vi "Define tração 90°C suporte.vi"(8 "error in (no error)":errorcluster, 11 "Dados SP":T1={"Condutor"={"Pc (N/m)"=0.0, "Mod.Young (N/m²)"=0.0, "Dil.Term.c (m/°C)"=0.0, "Área  (m²)"=0.0, "Tração EDS (N)"=0.0, "Tração Torig(N)"=0.0, "Tração Talta (N)"=0.0}, "Suporte"={"Ps (N/m)"=0.0, "Es (N/m²)"=0.0, "DTc (1/°C)"=0.0, "Área sup (m²)"=0.0, "Tração EDS sup (N)"=0.0, "Tração AT sup (N)"=0.0, "Flecha sup AT (m)"=0.0}, "Vão"={"Extensão (m)"=0.0, "Desnivel (m)"=0.0, "Flecha à 60 °C"=0.0}, "Projeto"={"Temp. EDS (°C)"=0.0, "Lim.original (°C)"=0.0, "Lim.extend. (°C)"=0.0, "N. cabo/fase"=1.0}, "Subvão"={"Ext.Lim (m)"=0.0, "N. Esp."=0.0, "F.lim (m)"=0.0, "Ext.calc"=0.0, "Ext.definido"=0.0, "Comp.cabo"=0.0, "Ext.55%"=0.0, "Tração sub\nAT (N)"=0.0, "Ext.sel."=0.0, "Flecha lim.\ncalc (m)"=0.0}, "Vetor de dados"={"Coor.X.esp"=[], "Coor.Y.Esp."=[], "Sub.vao X"=[], "Sub.vao Y"=[], "CoordY.sup"=[], "CoordX.sup"=[]}} {"Subvão"."Comp.cabo" min=1.0 max=8.0 step=1.0}) -> (0 "error out":errorcluster, 3 "Dados SP Out":T1={"Condutor"={"Pc (N/m)"=0.0, "Mod.Young (N/m²)"=0.0, "Dil.Term.c (m/°C)"=0.0, "Área  (m²)"=0.0, "Tração EDS (N)"=0.0, "Tração Torig(N)"=0.0, "Tração Talta (N)"=0.0}, "Suporte"={"Ps (N/m)"=0.0, "Es (N/m²)"=0.0, "DTc (1/°C)"=0.0, "Área sup (m²)"=0.0, "Tração EDS sup (N)"=0.0, "Tração AT sup (N)"=0.0, "Flecha sup AT (m)"=0.0}, "Vão"={"Extensão (m)"=0.0, "Desnivel (m)"=0.0, "Flecha à 60 °C"=0.0}, "Projeto"={"Temp. EDS (°C)"=0.0, "Lim.original (°C)"=0.0, "Lim.extend. (°C)"=0.0, "N. cabo/fase"=1.0}, "Subvão"={"Ext.Lim (m)"=0.0, "N. Esp."=0.0, "F.lim (m)"=0.0, "Ext.calc"=0.0, "Ext.definido"=0.0, "Comp.cabo"=0.0, "Ext.55%"=0.0, "Tração sub\nAT (N)"=0.0, "Ext.sel."=0.0, "Flecha lim.\ncalc (m)"=0.0}, "Vetor de dados"={"Coor.X.esp"=[], "Coor.Y.Esp."=[], "Sub.vao X"=[], "Sub.vao Y"=[], "CoordY.sup"=[], "CoordX.sup"=[]}} {"Subvão"."Comp.cabo" min=1.0 max=8.0 step=1.0})   [LabVIEW 2020]
uses:
  controls/SP data.ctl
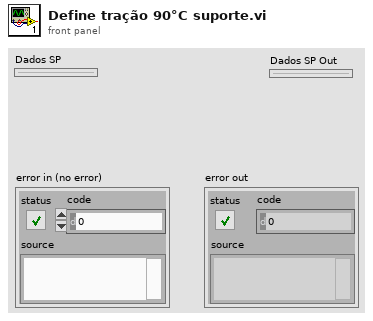
[diagram p1: front panel]
types:
  T1 = typedef "SP data.ctl" = cluster{"Condutor":cluster{"Pc (N/m)":dbl, "Mod.Young (N/m²)":dbl, "Dil.Term.c (m/°C)":dbl, "Área  (m²)":dbl, "Tração EDS (N)":dbl, "Tração Torig(N)":dbl, "Tração Talta (N)":dbl}, "Suporte":cluster{"Ps (N/m)":dbl, "Es (N/m²)":dbl, "DTc (1/°C)":dbl, "Área sup (m²)":dbl, "Tração EDS sup (N)":dbl, "Tração AT sup (N)":dbl, "Flecha sup AT (m)":dbl}, "Vão":cluster{"Extensão (m)":dbl, "Desnivel (m)":dbl, "Flecha à 60 °C":dbl}, "Projeto":cluster{"Temp. EDS (°C)":dbl, "Lim.original (°C)":dbl, "Lim.extend. (°C)":dbl, "N. cabo/fase":dbl}, "Subvão":cluster{"Ext.Lim (m)":dbl, "N. Esp.":dbl, "F.lim (m)":dbl, "Ext.calc":dbl, "Ext.definido":dbl, "Comp.cabo":dbl, "Ext.55%":dbl, "Tração sub\nAT (N)":dbl, "Ext.sel.":dbl, "Flecha lim.\ncalc (m)":dbl}, "Vetor de dados":cluster{"Coor.X.esp":dbl[], "Coor.Y.Esp.":dbl[], "Sub.vao X":dbl[], "Sub.vao Y":dbl[], "CoordY.sup":dbl[], "CoordX.sup":dbl[]}}
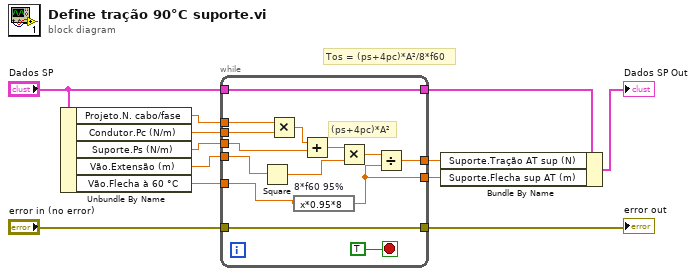
[diagram p0: block diagram]
diagram:
  # "Tos = (ps+4pc)*A²/8*f60"
  n1 = Unbundle By Name("Dados SP") -> ("Projeto.N. cabo/fase"=w6:dbl, "Condutor.Pc (N/m)"=w5:dbl, "Suporte.Ps (N/m)"=w4:dbl, "Vão.Extensão (m)"=w3:dbl, "Vão.Flecha à 60 °C"=w2:dbl)
  n2 = while {
    tunnel: "Dados SP" -> [w25]
    tunnel: [w25] -> w10
    tunnel: "error in (no error)" -> [w24]
    tunnel: [w24] -> w11
    tunnel: w6 -> [w19]
    tunnel: w5 -> [w18]
    tunnel: w4 -> [w17]
    tunnel: w3 -> [w16]
    tunnel: [w15] -> w8
    tunnel: w2 -> [w14]
    tunnel: [w13] -> w1
    stop <- TRUE stop-if-true
    # "(ps+4pc)*A²"
    n3 = Square(x=w16) -> (x^2=w21:dbl)
    n4 = Multiply(x=w19, y=w18) -> (x*y=w23:dbl)
    n5 = expression code="x*0.95*8" "8*f60 95%"(w14) -> (w13:dbl)
    n6 = Add(x=w23, y=w17) -> (x+y=w22:dbl)
    n7 = Multiply(x=w22, y=w21) -> (x*y=w20:dbl)
    n8 = Divide(x=w20, y=w13) -> (x/y=w15:dbl)
  }
  "error out" <- w11
  n9 = Bundle By Name(cluster=w10, "Suporte.Tração AT sup (N)"=w8, "Suporte.Flecha sup AT (m)"=w1) -> (→"Dados SP Out":T1)
